vi "设置启动参数.vi"(5 "数组":cluster{"String":string, "Value":u16}[](array[cluster]), 7 "MB通信方式选择":enum16{"串口", "TCP"}(ring), 8 "Error in":errorcluster caption="Error in (no error)", 9 "Port (502)":u16=502, 10 "IP Address":string="localhost", 11 "VISA Resource":refnum<visa-resource-name>) -> (0 "error out":errorcluster)   [LabVIEW 2016, in "斯坦道总磷.lvlib"]
uses:
  <vilib>/Plasmionique/MB Master/MB_Master_Serial/MB_Master_Serial.lvclass
  C:/Program Files (x86)/National Instruments/LabVIEW 2016/vi.lib/Plasmionique/MB Master/MB_Master/MB_Master.lvclass
  <vilib>/Plasmionique/MB Master/MB_Master_TCP/MB_Master_TCP.lvclass
  <vilib>/Plasmionique/MB Master/MB_Master/MB_Master.lvclass
  <vilib>/Plasmionique/MB Master/MB Master.lvlib
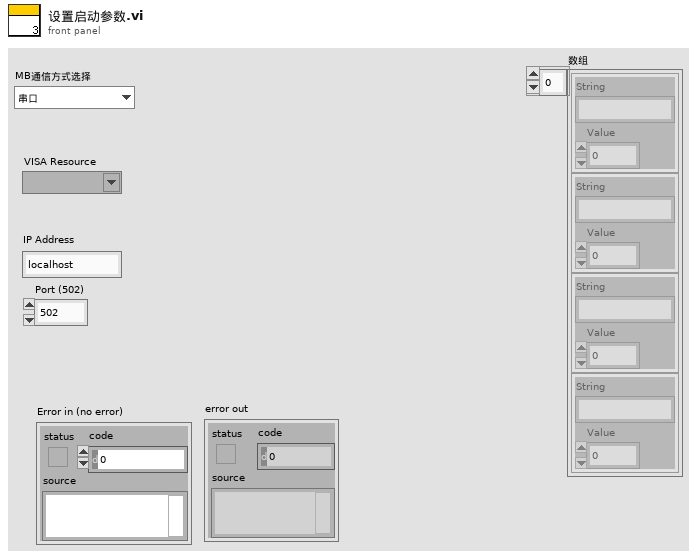
[diagram p1: front panel]
types:
  T1 = cluster{"baud rate (bps)":u32, "stop bits":u16, "parity":u16, "flow control":u16, "timeout":u32, "retries":i32}
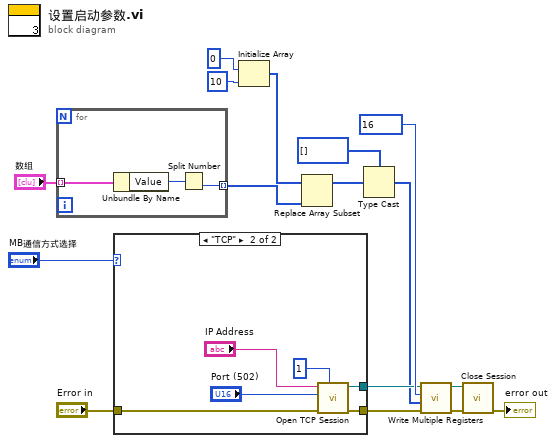
[diagram p0: block diagram]
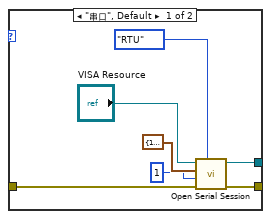
[diagram p2: hidden frame]
diagram:
  n1 = for {
    tunnel: "数组" -> [w19] mode=indexing
    tunnel: [w17] -> w4 mode=indexing
    n2 = Unbundle By Name(w19) -> ("Value"=w18:u16)
    n3 = Split Number(x=w18) -> (lo(x)=w17:u8)  [unwired: 1 out]
  }
  n4 = case shown="\"TCP\"" "MB通信方式选择" {
    tunnel: [w26 w32] -> w15
    tunnel: "Error in" -> [w21 w30]
    tunnel: [w20 w31] -> w12
    frame "串口", Default {
      n5 = call <vilib>:"Open Serial Session.vi"("Mode (RTU)"=enum16{"RTU", "ASCII"}."RTU", "Error in"=w21, "Slave ID"=u8 1, "Serial Config"=T1 {"baud rate (bps)"=115200, "stop bits"=10, "parity"=0, "flow control"=0, "timeout"=1000, "retries"=1}, "VISA Resource"="VISA Resource") -> ("Error out"=w20:errorcluster, "MB_Serial session"=w26:refnum<class "MB_Master_Serial.lvclass">)  [unwired: 5 in]
    }
    frame "TCP" {
      n6 = call <vilib>:"Open TCP Session.vi"("Slave ID (255)"=u8 1, "error in (no error)"=w30, "Port (502)"="Port (502)", "IP Address"="IP Address") -> ("error out"=w31:errorcluster, "MB_TCP session"=w32:refnum<class "MB_Master_TCP.lvclass">)  [unwired: 6 in]
    }
  }
  n7 = Initialize Array(u8 0, 10 ("维数大小")) -> (w5:u8[])
  n8 = Replace Array Subset(array=w5, new element=w4) -> (w3:u8[])  [unwired: 1 in]
  n9 = Type Cast(type=u16[] [], x=w3) -> (*(type *) &x=w1:u16[])
  n10 = call <vilib>:"Write Multiple Registers.vi"("error in (no error)"=w12, "values"=w1, "starting address"=u16 16, "MB session in"=w15) -> ("error out"=w11:errorcluster, "MB session out"=w14:refnum<class "MB_Master.lvclass">)  [unwired: 6 in]
  n11 = call-dynamic "Close Session.vi"("error in (no error)"=w11, "MB session in"=w14) -> ("error out"=→"error out":errorcluster)  [unwired: 9 in]
